vi "iitk.vi"() -> ()   [LabVIEW 2018]
uses:
  <vilib>/Waveform/WDTFileIO.llb/Read Waveform from File.vi
  <vilib>/express/express analysis/Spectral/Block/exnSpectralBlock spectral measurements peak poly.vi
  <vilib>/express/express analysis/Spectral/Block/exnSpectralBlock spectral measurements peak DDT.vi
  <vilib>/Waveform/WDTFileIO.llb/Export Waveforms To Spreadsheet File (1D).vi
  <vilib>/express/express analysis/Spectral/XNode/ExpressSpectralMeasurementsBlockNode.xnode
panel:
  in  "Operating Mode 3":T1(ring)=enum."Analyze Real-time"
  out "Orignal Signal 2":dynamicdata(graph)
  in  "Threshold 2":dbl=0.1
  out "Portion 2":dynamicdata(graph)
  in  "Portion Duration 2":i32=200
  out "Index 7":dbl
  out "Index 6":dbl
  out "Index 5":dbl
  out "Index 4":dbl
  out "dt1 2":dbl
  out "dt2 2":dbl
  out "dt3 2":dbl
  in  "Manual depth 2":dbl=4.3
  in  "Mode 2":T2(ring)=enum."Use Far Field"
  out "x 2":dbl format="%#_6f"
  out "y 2":dbl format="%#_6f"
  out "z 2":dbl
  in  "peak min 2":dbl=0.1
  out "ratio 8":dbl
  out "ratio 7":dbl
  out "ratio 6":dbl
  out "ratio 5":dbl
  out "amplitude 8":dbl
  out "amplitude 7":dbl
  out "amplitude 6":dbl
  out "amplitude 5":dbl
  out "yaw 2":dbl
  out "pitch 2":dbl
  out "Yaw Chart 2":dbl(graph)
  out "Freq Domain 2":dynamicdata(graph)
  out "Ratio at Index (%) 2":dbl
  in  "LPF Cut-Off 2":dbl=40000.0 caption="Lower Cut-Off"
  out "Selected Index 2":i32
  in  "method":bool
  in  "file path (dialog if empty)":path
  in  "Operating Mode 2":T1(ring)=enum."Analyze Real-time"
  out "Orignal Signal":dynamicdata(graph)
  in  "Threshold":dbl=0.1
  out "Portion":dynamicdata(graph)
  in  "Portion Duration":i32=200
  out "Index 0":dbl
  out "Index 1":dbl
  out "Index 2":dbl
  out "Index 3":dbl
  out "dt1":dbl
  out "dt2":dbl
  out "dt3":dbl
  in  "Manual depth":dbl=4.3
  in  "Mode":T2(ring)=enum."Use Far Field"
  out "x":dbl format="%#_6f"
  out "y":dbl format="%#_6f"
  out "z":dbl
  in  "peak min":dbl=0.1
  out "ratio":dbl
  out "ratio 2":dbl
  out "ratio 3":dbl
  out "ratio 4":dbl
  out "amplitude":dbl
  out "amplitude 2":dbl
  out "amplitude 3":dbl
  out "amplitude 4":dbl
  out "yaw":dbl
  out "pitch":dbl
  out "Yaw Chart":dbl(graph)
  out "Freq Domain":dynamicdata(graph)
  out "Ratio at Index (%)":dbl
  in  "LPF Cut-Off":dbl=40000.0 caption="Lower Cut-Off"
  out "Selected Index":i32
  in  "stop (F)":bool
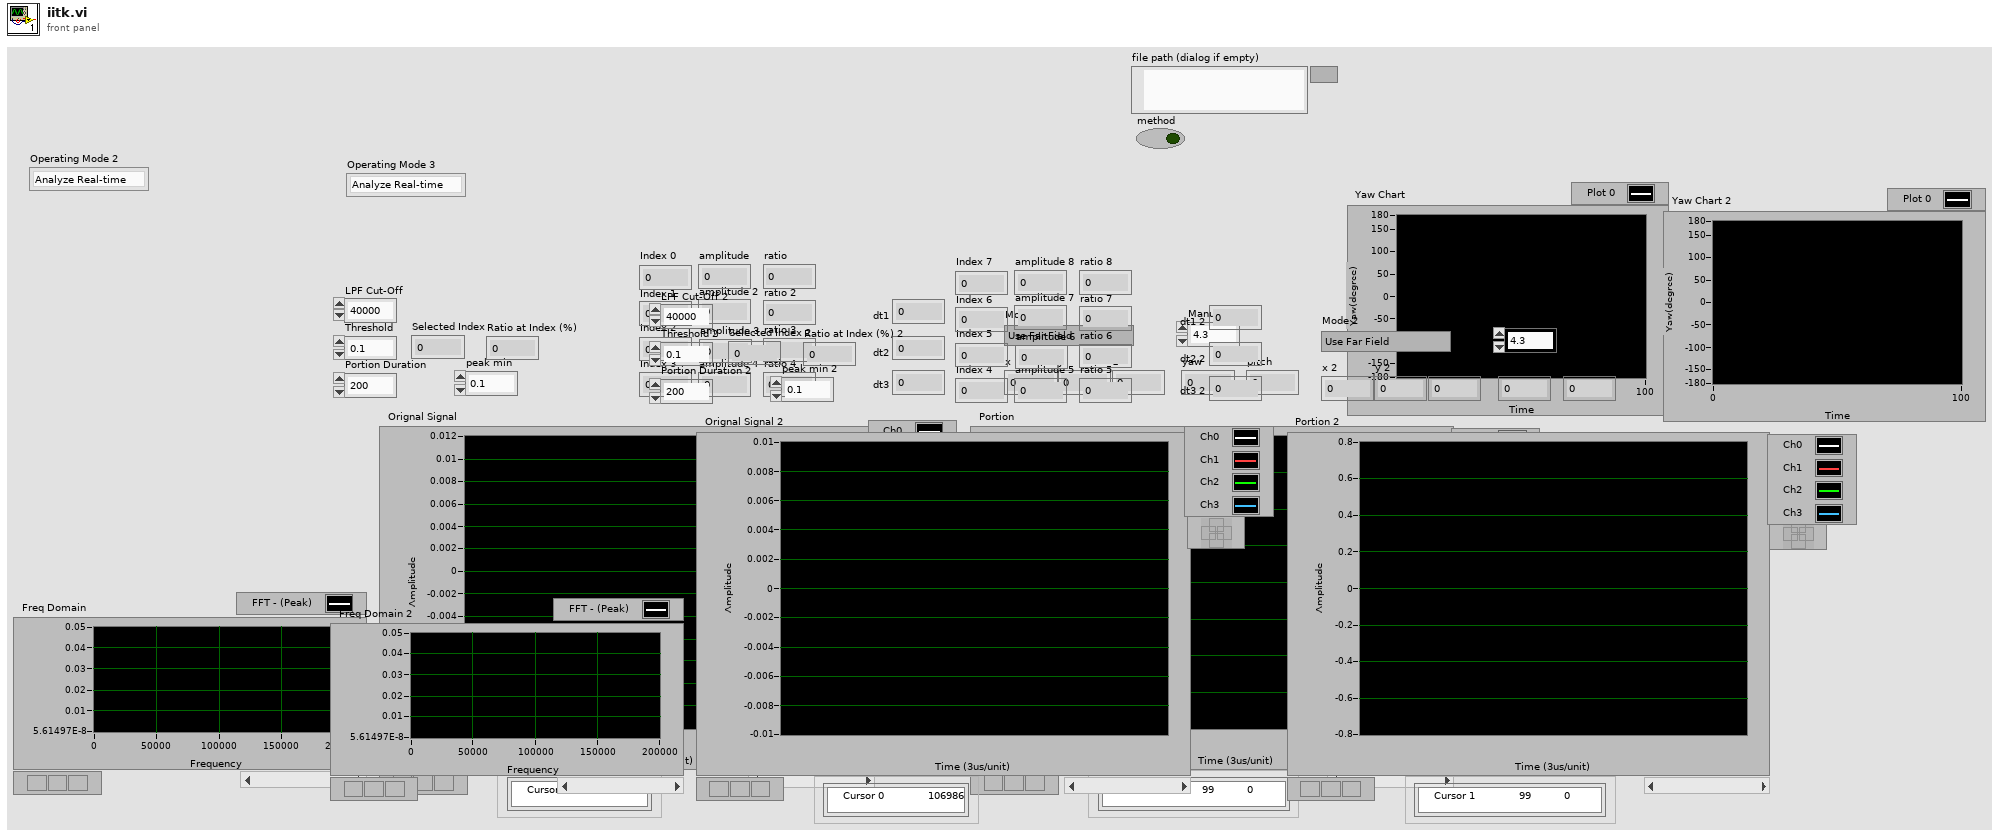
[diagram p1: front panel]
types:
  T1 = enum16{"Analyze From File", "Record Data", "Analyze Real-time"}
  T2 = enum16{"Use Near Field", "Use Far Field", "Send to ROS", "Far Field with 3 hydrophones"}
  T3 = cluster{"averaging mode":u16, "weighting mode":u16, "number of averages":u32}
  T4 = cluster{"dB On (F)":bool, "unwrap phase (F)":bool, "convert to degree (F)":bool}
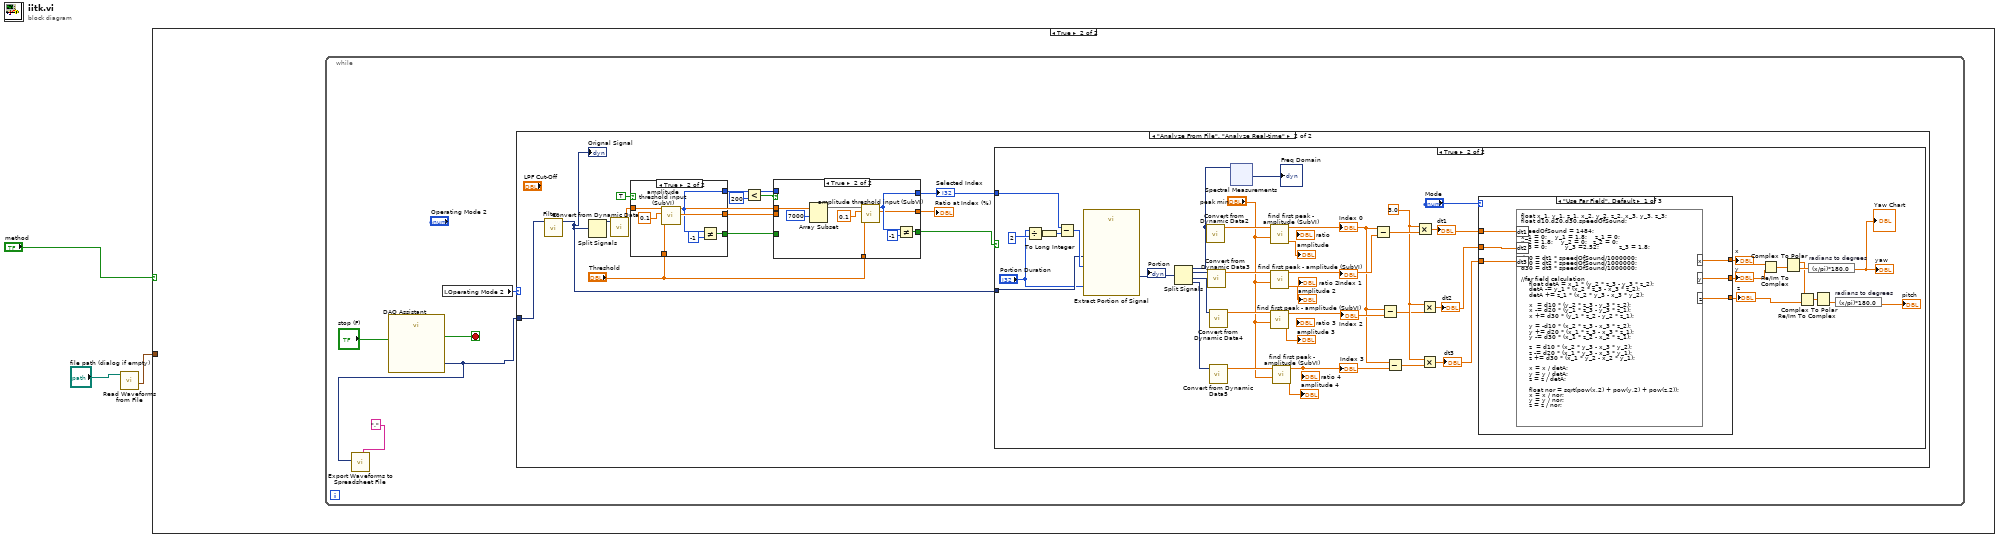
[diagram p0: block diagram]
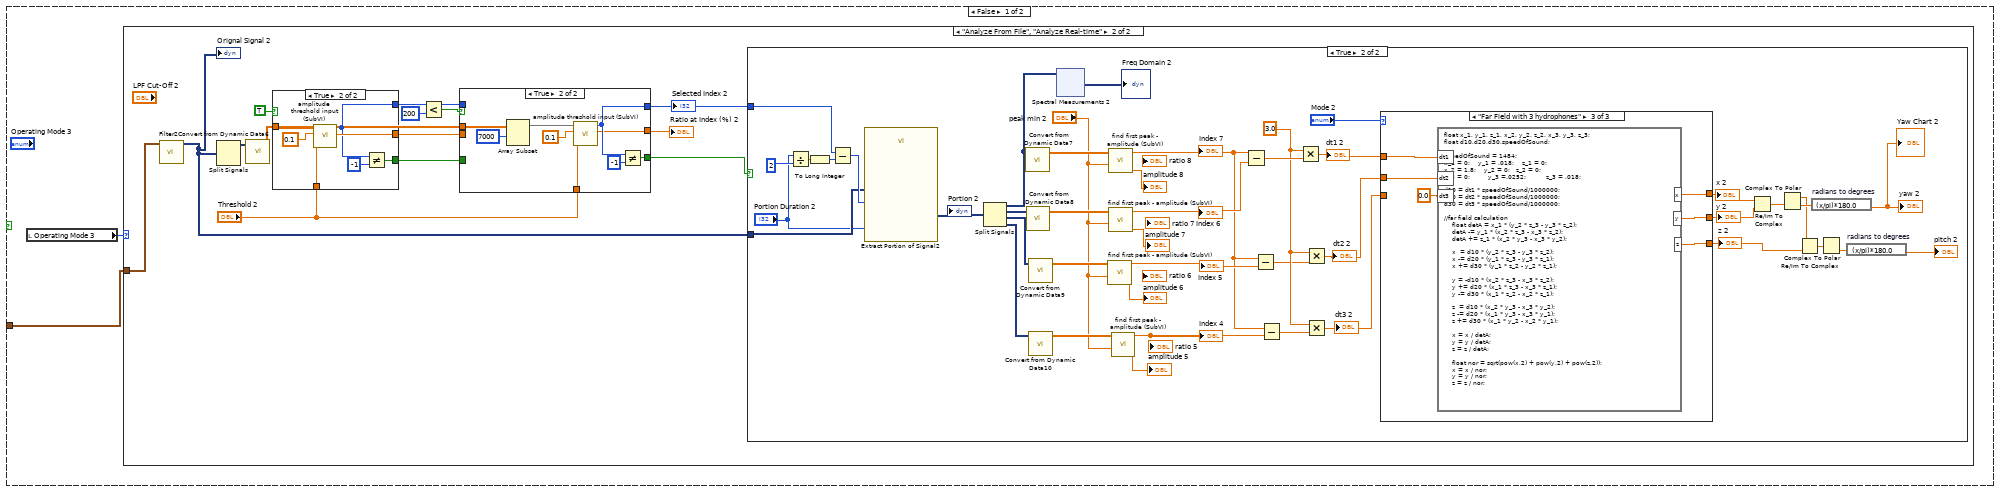
[diagram p2: hidden frame]
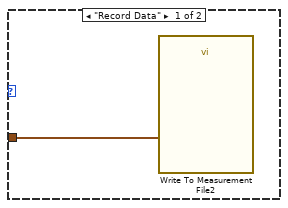
[diagram p3: hidden frame]
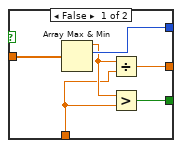
[diagram p5: hidden frame]
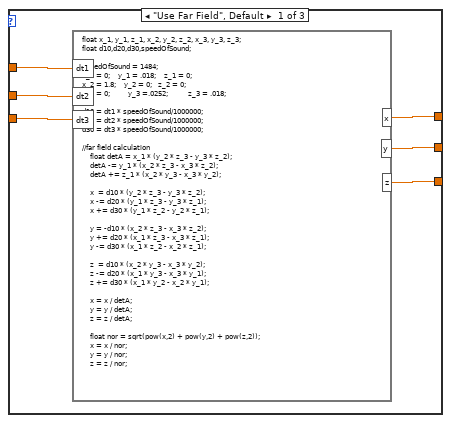
[diagram p7: hidden frame]
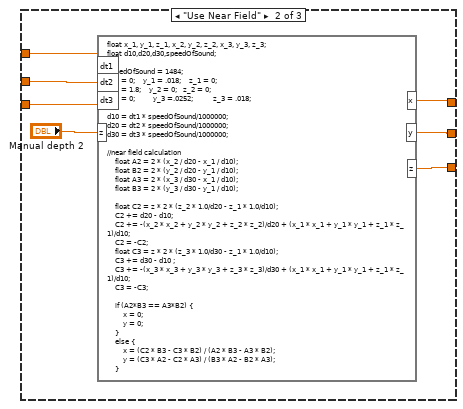
[diagram p8: hidden frame]
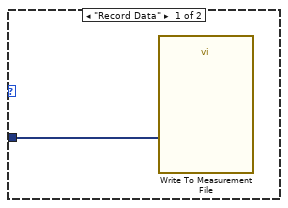
[diagram p9: hidden frame]
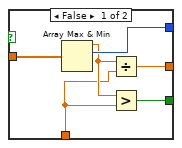
[diagram p11: hidden frame]
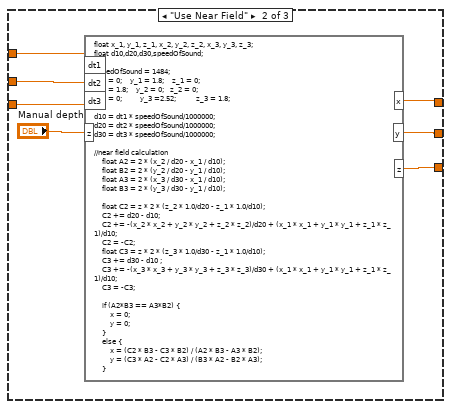
[diagram p13: hidden frame]
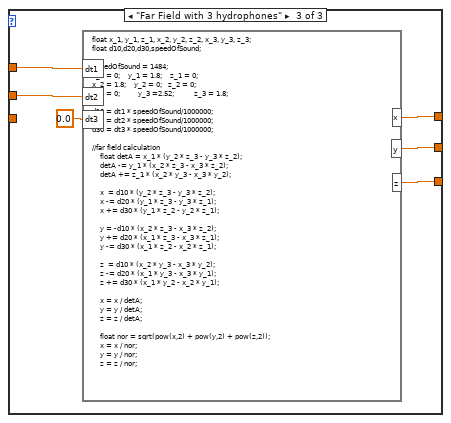
[diagram p14: hidden frame]
diagram:
  n1 = call-poly <vilib>:"Read Waveforms from File.vi"("file path (dialog if empty)"="file path (dialog if empty)") -> ("all waveforms in record"=w1:waveform(dbl)[])  [unwired: 5 in, 3 out]
  n2 = case shown="True" "method" {
    tunnel: w1 -> [w4 _]
    frame False {
      n3 = local read "Operating Mode 3"() -> (w5:T1)
      n4 = case shown="\"Analyze From File\", \"Analyze Real-time\"" w5 {
        tunnel: w4 -> [w6 w9]
        frame "Record Data" {
          n5 = call "Write To Measurement File2"("Signals"=w6) -> ()  [unwired: 16 in, 3 out]
        }
        frame "Analyze From File", "Analyze Real-time" {
          n6 = call "Filter2"("Signal"=w9) -> ("Filtered Signal"=w7:dynamicdata)  [unwired: 9 in, 1 out]
          "Orignal Signal 2" <- w7
          n7 = Split Signals(w7) -> (w8:dynamicdata)  [unwired: 4 in, 3 out]
          n8 = call "Convert from Dynamic Data6"("Dynamic Data Type"=w8) -> ("Array"=w15:dbl[])  [unwired: 3 in]
          n9 = case shown="True" TRUE {
            tunnel: w15 -> [w38 w45]
            tunnel: [w35 w42] -> w16
            tunnel: [w36 w41] -> w11
            tunnel: [w37 w40] -> w19
            tunnel: "Threshold 2" -> [w33 w39]
            frame False {
              n10 = Array Max & Min(array=w38) -> (max value=w34:dbl, max index (indices)=w36:i32)  [unwired: 2 out]
              n11 = Divide(x=w34, y=w33) -> (x/y=w35:dbl)
              n12 = Greater?(x=w34, y=w33) -> (0:w37:bool)
            }
            frame True {
              n13 = call "amplitude threshold input (SubVI).vi"("threshold"=w39, "%max amplitude"=0.1, "Array"=w45) -> ("actual ratio (%)"=w42:dbl, "Index"=w41:i32)  [unwired: 7 in]
              n14 = Not Equal?(x=w41, y=-1) -> (x != y?=w40:bool)
            }
          }
          n15 = Less?(x=w11, y=200) -> (x < y?=w17:bool)
          n16 = case shown="True" w17 {
            tunnel: w19 -> [w23 _]
            tunnel: w16 -> [w21 _]
            tunnel: w15 -> [_ w32]
            tunnel: "Threshold 2" -> [_ w27]
            tunnel: [w23 w26] -> w13
            tunnel: [w22 w25] -> w10
            tunnel: [w21 w24] -> w12
            tunnel: w11 -> [w22 _]
            frame False {
            }
            frame True {
              n17 = Array Subset(array=w32, index=7000) -> (w28:dbl[])  [unwired: 1 in]
              n18 = call "amplitude threshold input (SubVI).vi"("threshold"=w27, "%max amplitude"=0.1, "Array"=w28) -> ("actual ratio (%)"=w24:dbl, "Index"=w25:i32)  [unwired: 7 in]
              n19 = Not Equal?(x=w25, y=-1) -> (x != y?=w26:bool)
            }
          }
          "Ratio at Index (%) 2" <- w12
          "Selected Index 2" <- w10
          n20 = case shown="True" w13 {
            tunnel: w7 -> [_ w86]
            tunnel: w10 -> [_ w52]
            frame False {
            }
            frame True {
              w82 = 3.0 ("x")
              n21 = Divide(x="Portion Duration 2", y=2) -> (x/y=w56:dbl)
              n22 = To Long Integer(number=w56) -> (32bit integer=w55:i32)
              n23 = Subtract(x=w52, y=w55) -> (x-y=w89:i32)
              n24 = call "Extract Portion of Signal2"("Samples"="Portion Duration 2", "Begin Sample"=w89, "Signals"=w86) -> ("Section"=w85:dynamicdata)  [unwired: 7 in, 1 out]
              "Portion 2" <- w85
              n25 = Split Signals(w85) -> (w46:dynamicdata, w88:dynamicdata, w87:dynamicdata, w84:dynamicdata)  [unwired: 4 in]
              n26 = call "Convert from Dynamic Data7"("Dynamic Data Type"=w46) -> ("Array"=w77:dbl[])  [unwired: 3 in]
              n27 = call "Convert from Dynamic Data8"("Dynamic Data Type"=w88) -> ("Array"=w76:dbl[])  [unwired: 3 in]
              n28 = call "Convert from Dynamic Data9"("Dynamic Data Type"=w87) -> ("Array"=w75:dbl[])  [unwired: 3 in]
              n29 = call "Convert from Dynamic Data10"("Dynamic Data Type"=w84) -> ("Array"=w74:dbl[])  [unwired: 3 in]
              n30 = xnode "Spectral Measurements 2"("Signals"=w46) -> ("FFT - (Peak)"=→"Freq Domain 2":dynamicdata)  [unwired: 1 in, 2 out]
              n31 = call "find first peak - amplitude (SubVI).vi"("threshold ratio"="peak min 2", "Array"=w75) -> ("Peak threshold"=→"amplitude 6":dbl, "Index"=w72:dbl)  [unwired: 5 in, 3 out]
              "Index 5" <- w72
              n32 = call "find first peak - amplitude (SubVI).vi"("threshold ratio"="peak min 2", "Array"=w77) -> ("Peak threshold"=→"amplitude 8":dbl, "Index"=w71:dbl)  [unwired: 5 in, 3 out]
              "Index 7" <- w71
              n33 = call "find first peak - amplitude (SubVI).vi"("threshold ratio"="peak min 2", "Array"=w76) -> ("Peak threshold"=→"amplitude 7":dbl, "Index"=w73:dbl)  [unwired: 5 in, 3 out]
              "Index 6" <- w73
              n34 = call "find first peak - amplitude (SubVI).vi"("threshold ratio"="peak min 2", "Array"=w74) -> ("Peak threshold"=→"amplitude 5":dbl, "Index"=w70:dbl)  [unwired: 5 in, 3 out]
              "Index 4" <- w70
              n35 = Subtract(x=w71, y=w73) -> (x-y=w83:dbl)
              n36 = Subtract(x=w71, y=w72) -> (x-y=w81:dbl)
              n37 = Subtract(x=w71, y=w70) -> (x-y=w80:dbl)
              n38 = Multiply(x=w82, y=w83) -> (x*y=w59:dbl)
              "dt1 2" <- w59
              n39 = Multiply(x=w82, y=w81) -> (x*y=w79:dbl)
              "dt2 2" <- w79
              n40 = Multiply(x=w82, y=w80) -> (x*y=w58:dbl)
              "dt3 2" <- w58
              n41 = case shown="\"Far Field with 3 hydrophones\"" "Mode 2" {
                tunnel: w59 -> [w105 w112 w118]
                tunnel: w79 -> [w104 w111 w117]
                tunnel: [w103 w110 w115] -> w66
                tunnel: [w102 w109 w114] -> w65
                tunnel: [w101 w108 w113] -> w64
                tunnel: w58 -> [w100 w106 _]
                frame "Use Far Field", Default {
                  n42 = formula code="float x_1, y_1, z_1, x_2, y_2, z_2, x_3, y_3, z_3;\nfloat d10,d20,d30,speedOfSound;\n\nspeedOfSound = 1484;\nx_1 = 0;    y_1 = .018;    z_1 = 0;\nx_2 = 1.8;    y_2 = 0;   z_2 = 0;\nx_3 = 0;         y_3 =.0252;          z_3 = .018;\n\nd10 = dt1 * speedOfSound/1000000;\nd20 = dt2 * speedOfSound/1000000;\nd30 = dt3 * speedOfSound/1000000;\n\n//far field calculation\n    float detA = x_1 * (y_2 * z_3 - y_3 * z_2);\n    detA -= y_1 * (x_2 * z_3 - x_3 * z_2);\n    detA += z_1 * (x_2 * y_3 - x_3 * y_2);\n\n    x  = d10 * (y_2 * z_3 - y_3 * z_2);\n    x -= d20 * (y_1 * z_3 - y_3 * z_1);\n    x += d30 * (y_1 * z_2 - y_2 * z_1);\n\n    y = -d10 * (x_2 * z_3 - x_3 * z_2);\n    y += d20 * (x_1 * z_3 - x_3 * z_1);\n    y -= d30 * (x_1 * z_2 - x_2 * z_1);\n\n    z  = d10 * (x_2 * y_3 - x_3 * y_2);\n    z -= d20 * (x_1 * y_3 - x_3 * y_1);\n    z += d30 * (x_1 * y_2 - x_2 * y_1);\n\n    x = x / detA;\n    y = y / detA;\n    z = z / detA;\n\n    float nor = sqrt(pow(x,2) + pow(y,2) + pow(z,2));\n    x = x / nor;\n    y = y / nor;\n    z = z / nor;"("dt1"=w105, "dt2"=w104, "dt3"=w100) -> ("x"=w103:dbl, "y"=w102:dbl, "z"=w101:dbl)
                }
                frame "Use Near Field" {
                  n43 = formula code="float x_1, y_1, z_1, x_2, y_2, z_2, x_3, y_3, z_3;\nfloat d10,d20,d30,speedOfSound;\n\nspeedOfSound = 1484;\nx_1 = 0;    y_1 = .018;    z_1 = 0;\nx_2 = 1.8;    y_2 = 0;   z_2 = 0;\nx_3 = 0;         y_3 =.0252;          z_3 = .018;\n\nd10 = dt1 * speedOfSound/1000000;\nd20 = dt2 * speedOfSound/1000000;\nd30 = dt3 * speedOfSound/1000000;\n\n//near field calculation\n    float A2 = 2 * (x_2 / d20 - x_1 / d10);\n    float B2 = 2 * (y_2 / d20 - y_1 / d10);\n    float A3 = 2 * (x_3 / d30 - x_1 / d10);\n    float B3 = 2 * (y_3 / d30 - y_1 / d10);\n    \n    float C2 = z * 2 * (z_2 * 1.0/d20 - z_1 * 1.0/d10);\n    C2 += d20 - d10;\n    C2 += -(x_2 * x_2 + y_2 * y_2 + z_2 * z_2)/d20 + (x_1 * x_1 + y_1 * y_1 + z_1 * z_1)/d10;\n    C2 = -C2;\n    float C3 = z * 2 * (z_3 * 1.0/d30 - z_1 * 1.0/d10);\n    C3 += d30 - d10 ;\n    C3 += -(x_3 * x_3 + y_3 * y_3 + z_3 * z_3)/d30 + (x_1 * x_1 + y_1 * y_1 + z_1 * z_1)/d10;\n    C3 = -C3;\n\n    if (A2*B3 == A3*B2) {\n        x = 0;\n        y = 0;\n    }\n    else {\n        x = (C2 * B3 - C3 * B2) / (A2 * B3 - A3 * B2);\n        y = (C3 * A2 - C2 * A3) / (B3 * A2 - B2 * A3);\n    }"("dt1"=w112, "dt2"=w111, "dt3"=w106, "z"="Manual depth 2") -> ("x"=w110:dbl, "y"=w109:dbl, "z"=w108:dbl)
                }
                frame "Far Field with 3 hydrophones" {
                  n44 = formula code="float x_1, y_1, z_1, x_2, y_2, z_2, x_3, y_3, z_3;\nfloat d10,d20,d30,speedOfSound;\n\nspeedOfSound = 1484;\nx_1 = 0;    y_1 = .018;    z_1 = 0;\nx_2 = 1.8;    y_2 = 0;   z_2 = 0;\nx_3 = 0;         y_3 =.0252;          z_3 = .018;\n\nd10 = dt1 * speedOfSound/1000000;\nd20 = dt2 * speedOfSound/1000000;\nd30 = dt3 * speedOfSound/1000000;\n\n//far field calculation\n    float detA = x_1 * (y_2 * z_3 - y_3 * z_2);\n    detA -= y_1 * (x_2 * z_3 - x_3 * z_2);\n    detA += z_1 * (x_2 * y_3 - x_3 * y_2);\n\n    x  = d10 * (y_2 * z_3 - y_3 * z_2);\n    x -= d20 * (y_1 * z_3 - y_3 * z_1);\n    x += d30 * (y_1 * z_2 - y_2 * z_1);\n\n    y = -d10 * (x_2 * z_3 - x_3 * z_2);\n    y += d20 * (x_1 * z_3 - x_3 * z_1);\n    y -= d30 * (x_1 * z_2 - x_2 * z_1);\n\n    z  = d10 * (x_2 * y_3 - x_3 * y_2);\n    z -= d20 * (x_1 * y_3 - x_3 * y_1);\n    z += d30 * (x_1 * y_2 - x_2 * y_1);\n\n    x = x / detA;\n    y = y / detA;\n    z = z / detA;\n\n    float nor = sqrt(pow(x,2) + pow(y,2) + pow(z,2));\n    x = x / nor;\n    y = y / nor;\n    z = z / nor;"("dt1"=w118, "dt2"=w117, "dt3"=0.0 ("input variable")) -> ("x"=w115:dbl, "y"=w114:dbl, "z"=w113:dbl)
                }
              }
              "x 2" <- w66
              "y 2" <- w65
              "z 2" <- w64
              n45 = Re/Im To Complex(1:w65, 2:w66) -> (0:w68:cdb)
              n46 = Complex To Polar(r * e^(i*theta)=w68) -> (r=w63:dbl, theta=w67:dbl)
              n47 = Re/Im To Complex(1:w64, 2:w63) -> (0:w62:cdb)
              n48 = expression code="(x/pi)*180.0" "radians to degrees"(w67) -> (→"yaw 2" →"Yaw Chart 2":dbl)
              n49 = Complex To Polar(r * e^(i*theta)=w62) -> (theta=w60:dbl)  [unwired: 1 out]
              n50 = expression code="(x/pi)*180.0" "radians to degrees"(w60) -> (→"pitch 2":dbl)
            }
          }
        }
      }
    }
    frame True {
      n51 = while {
        stop <- w123 stop-if-true
        n52 = call "DAQ Assistant"("stop (F)"="stop (F)") -> ("data"=w119:dynamicdata, "stopped"=w123:bool)  [unwired: 15 in, 2 out]
        n53 = call-poly <vilib>:"Export Waveforms to Spreadsheet File.vi"("delimiter (Tab)"=".", "waveforms"=w119) -> ()  [unwired: 8 in, 2 out]
        n54 = local read "Operating Mode 2"() -> (w121:T1)
        n55 = case shown="\"Analyze From File\", \"Analyze Real-time\"" w121 {
          tunnel: w119 -> [w124 w127]
          frame "Record Data" {
            n56 = call "Write To Measurement File"("Signals"=w124) -> ()  [unwired: 16 in, 3 out]
          }
          frame "Analyze From File", "Analyze Real-time" {
            n57 = call "Filter"("Signal"=w127) -> ("Filtered Signal"=w125:dynamicdata)  [unwired: 9 in, 1 out]
            "Orignal Signal" <- w125
            n58 = Split Signals(w125) -> (w126:dynamicdata)  [unwired: 4 in, 3 out]
            n59 = call "Convert from Dynamic Data"("Dynamic Data Type"=w126) -> ("Array"=w133:dbl[])  [unwired: 3 in]
            n60 = case shown="True" TRUE {
              tunnel: w133 -> [w156 w163]
              tunnel: [w153 w160] -> w134
              tunnel: [w154 w159] -> w129
              tunnel: [w155 w158] -> w137
              tunnel: "Threshold" -> [w151 w157]
              frame False {
                n61 = Array Max & Min(array=w156) -> (max value=w152:dbl, max index (indices)=w154:i32)  [unwired: 2 out]
                n62 = Divide(x=w152, y=w151) -> (x/y=w153:dbl)
                n63 = Greater?(x=w152, y=w151) -> (0:w155:bool)
              }
              frame True {
                n64 = call "amplitude threshold input (SubVI).vi"("threshold"=w157, "%max amplitude"=0.1, "Array"=w163) -> ("actual ratio (%)"=w160:dbl, "Index"=w159:i32)  [unwired: 7 in]
                n65 = Not Equal?(x=w159, y=-1) -> (x != y?=w158:bool)
              }
            }
            n66 = Less?(x=w129, y=200) -> (x < y?=w135:bool)
            n67 = case shown="True" w135 {
              tunnel: w137 -> [w141 _]
              tunnel: w134 -> [w139 _]
              tunnel: w133 -> [_ w150]
              tunnel: "Threshold" -> [_ w145]
              tunnel: [w141 w144] -> w131
              tunnel: [w140 w143] -> w128
              tunnel: [w139 w142] -> w130
              tunnel: w129 -> [w140 _]
              frame False {
              }
              frame True {
                n68 = Array Subset(array=w150, index=7000) -> (w146:dbl[])  [unwired: 1 in]
                n69 = call "amplitude threshold input (SubVI).vi"("threshold"=w145, "%max amplitude"=0.1, "Array"=w146) -> ("actual ratio (%)"=w142:dbl, "Index"=w143:i32)  [unwired: 7 in]
                n70 = Not Equal?(x=w143, y=-1) -> (x != y?=w144:bool)
              }
            }
            "Ratio at Index (%)" <- w130
            "Selected Index" <- w128
            n71 = case shown="True" w131 {
              tunnel: w125 -> [_ w204]
              tunnel: w128 -> [_ w170]
              frame False {
              }
              frame True {
                w200 = 3.0 ("x")
                n72 = Divide(x="Portion Duration", y=2) -> (x/y=w174:dbl)
                n73 = To Long Integer(number=w174) -> (32bit integer=w173:i32)
                n74 = Subtract(x=w170, y=w173) -> (x-y=w207:i32)
                n75 = call "Extract Portion of Signal"("Samples"="Portion Duration", "Begin Sample"=w207, "Signals"=w204) -> ("Section"=w203:dynamicdata)  [unwired: 7 in, 1 out]
                "Portion" <- w203
                n76 = Split Signals(w203) -> (w164:dynamicdata, w206:dynamicdata, w205:dynamicdata, w202:dynamicdata)  [unwired: 4 in]
                n77 = call "Convert from Dynamic Data2"("Dynamic Data Type"=w164) -> ("Array"=w195:dbl[])  [unwired: 3 in]
                n78 = call "Convert from Dynamic Data3"("Dynamic Data Type"=w206) -> ("Array"=w194:dbl[])  [unwired: 3 in]
                n79 = call "Convert from Dynamic Data4"("Dynamic Data Type"=w205) -> ("Array"=w193:dbl[])  [unwired: 3 in]
                n80 = call "Convert from Dynamic Data5"("Dynamic Data Type"=w202) -> ("Array"=w192:dbl[])  [unwired: 3 in]
                n81 = xnode "Spectral Measurements"("Signals"=w164) -> ("FFT - (Peak)"=→"Freq Domain":dynamicdata)  [unwired: 1 in, 2 out]
                n82 = call "find first peak - amplitude (SubVI).vi"("threshold ratio"="peak min", "Array"=w193) -> ("Peak threshold"=→"amplitude 3":dbl, "Index"=w190:dbl)  [unwired: 5 in, 3 out]
                "Index 2" <- w190
                n83 = call "find first peak - amplitude (SubVI).vi"("threshold ratio"="peak min", "Array"=w195) -> ("Peak threshold"=→"amplitude":dbl, "Index"=w189:dbl)  [unwired: 5 in, 3 out]
                "Index 0" <- w189
                n84 = call "find first peak - amplitude (SubVI).vi"("threshold ratio"="peak min", "Array"=w194) -> ("Peak threshold"=→"amplitude 2":dbl, "Index"=w191:dbl)  [unwired: 5 in, 3 out]
                "Index 1" <- w191
                n85 = call "find first peak - amplitude (SubVI).vi"("threshold ratio"="peak min", "Array"=w192) -> ("Peak threshold"=→"amplitude 4":dbl, "Index"=w188:dbl)  [unwired: 5 in, 3 out]
                "Index 3" <- w188
                n86 = Subtract(x=w189, y=w191) -> (x-y=w201:dbl)
                n87 = Subtract(x=w189, y=w190) -> (x-y=w199:dbl)
                n88 = Subtract(x=w189, y=w188) -> (x-y=w198:dbl)
                n89 = Multiply(x=w200, y=w201) -> (x*y=w177:dbl)
                "dt1" <- w177
                n90 = Multiply(x=w200, y=w199) -> (x*y=w197:dbl)
                "dt2" <- w197
                n91 = Multiply(x=w200, y=w198) -> (x*y=w176:dbl)
                "dt3" <- w176
                n92 = case shown="\"Use Far Field\", Default" "Mode" {
                  tunnel: w177 -> [w223 w230 w236]
                  tunnel: w197 -> [w222 w229 w235]
                  tunnel: [w221 w228 w233] -> w184
                  tunnel: [w220 w227 w232] -> w183
                  tunnel: [w219 w226 w231] -> w182
                  tunnel: w176 -> [w218 w224 _]
                  frame "Use Far Field", Default {
                    n93 = formula code="float x_1, y_1, z_1, x_2, y_2, z_2, x_3, y_3, z_3;\nfloat d10,d20,d30,speedOfSound;\n\nspeedOfSound = 1484;\nx_1 = 0;    y_1 = 1.8;    z_1 = 0;\nx_2 = 1.8;    y_2 = 0;   z_2 = 0;\nx_3 = 0;         y_3 =2.52;          z_3 = 1.8;\n\nd10 = dt1 * speedOfSound/1000000;\nd20 = dt2 * speedOfSound/1000000;\nd30 = dt3 * speedOfSound/1000000;\n\n//far field calculation\n    float detA = x_1 * (y_2 * z_3 - y_3 * z_2);\n    detA -= y_1 * (x_2 * z_3 - x_3 * z_2);\n    detA += z_1 * (x_2 * y_3 - x_3 * y_2);\n\n    x  = d10 * (y_2 * z_3 - y_3 * z_2);\n    x -= d20 * (y_1 * z_3 - y_3 * z_1);\n    x += d30 * (y_1 * z_2 - y_2 * z_1);\n\n    y = -d10 * (x_2 * z_3 - x_3 * z_2);\n    y += d20 * (x_1 * z_3 - x_3 * z_1);\n    y -= d30 * (x_1 * z_2 - x_2 * z_1);\n\n    z  = d10 * (x_2 * y_3 - x_3 * y_2);\n    z -= d20 * (x_1 * y_3 - x_3 * y_1);\n    z += d30 * (x_1 * y_2 - x_2 * y_1);\n\n    x = x / detA;\n    y = y / detA;\n    z = z / detA;\n\n    float nor = sqrt(pow(x,2) + pow(y,2) + pow(z,2));\n    x = x / nor;\n    y = y / nor;\n    z = z / nor;"("dt1"=w223, "dt2"=w222, "dt3"=w218) -> ("x"=w221:dbl, "y"=w220:dbl, "z"=w219:dbl)
                  }
                  frame "Use Near Field" {
                    n94 = formula code="float x_1, y_1, z_1, x_2, y_2, z_2, x_3, y_3, z_3;\nfloat d10,d20,d30,speedOfSound;\n\nspeedOfSound = 1484;\nx_1 = 0;    y_1 = 1.8;    z_1 = 0;\nx_2 = 1.8;    y_2 = 0;   z_2 = 0;\nx_3 = 0;         y_3 =2.52;          z_3 = 1.8;\n\nd10 = dt1 * speedOfSound/1000000;\nd20 = dt2 * speedOfSound/1000000;\nd30 = dt3 * speedOfSound/1000000;\n\n//near field calculation\n    float A2 = 2 * (x_2 / d20 - x_1 / d10);\n    float B2 = 2 * (y_2 / d20 - y_1 / d10);\n    float A3 = 2 * (x_3 / d30 - x_1 / d10);\n    float B3 = 2 * (y_3 / d30 - y_1 / d10);\n    \n    float C2 = z * 2 * (z_2 * 1.0/d20 - z_1 * 1.0/d10);\n    C2 += d20 - d10;\n    C2 += -(x_2 * x_2 + y_2 * y_2 + z_2 * z_2)/d20 + (x_1 * x_1 + y_1 * y_1 + z_1 * z_1)/d10;\n    C2 = -C2;\n    float C3 = z * 2 * (z_3 * 1.0/d30 - z_1 * 1.0/d10);\n    C3 += d30 - d10 ;\n    C3 += -(x_3 * x_3 + y_3 * y_3 + z_3 * z_3)/d30 + (x_1 * x_1 + y_1 * y_1 + z_1 * z_1)/d10;\n    C3 = -C3;\n\n    if (A2*B3 == A3*B2) {\n        x = 0;\n        y = 0;\n    }\n    else {\n        x = (C2 * B3 - C3 * B2) / (A2 * B3 - A3 * B2);\n        y = (C3 * A2 - C2 * A3) / (B3 * A2 - B2 * A3);\n    }"("dt1"=w230, "dt2"=w229, "dt3"=w224, "z"="Manual depth") -> ("x"=w228:dbl, "y"=w227:dbl, "z"=w226:dbl)
                  }
                  frame "Far Field with 3 hydrophones" {
                    n95 = formula code="float x_1, y_1, z_1, x_2, y_2, z_2, x_3, y_3, z_3;\nfloat d10,d20,d30,speedOfSound;\n\nspeedOfSound = 1484;\nx_1 = 0;    y_1 = 1.8;    z_1 = 0;\nx_2 = 1.8;    y_2 = 0;   z_2 = 0;\nx_3 = 0;         y_3 =2.52;          z_3 = 1.8;\n\nd10 = dt1 * speedOfSound/1000000;\nd20 = dt2 * speedOfSound/1000000;\nd30 = dt3 * speedOfSound/1000000;\n\n//far field calculation\n    float detA = x_1 * (y_2 * z_3 - y_3 * z_2);\n    detA -= y_1 * (x_2 * z_3 - x_3 * z_2);\n    detA += z_1 * (x_2 * y_3 - x_3 * y_2);\n\n    x  = d10 * (y_2 * z_3 - y_3 * z_2);\n    x -= d20 * (y_1 * z_3 - y_3 * z_1);\n    x += d30 * (y_1 * z_2 - y_2 * z_1);\n\n    y = -d10 * (x_2 * z_3 - x_3 * z_2);\n    y += d20 * (x_1 * z_3 - x_3 * z_1);\n    y -= d30 * (x_1 * z_2 - x_2 * z_1);\n\n    z  = d10 * (x_2 * y_3 - x_3 * y_2);\n    z -= d20 * (x_1 * y_3 - x_3 * y_1);\n    z += d30 * (x_1 * y_2 - x_2 * y_1);\n\n    x = x / detA;\n    y = y / detA;\n    z = z / detA;\n\n    float nor = sqrt(pow(x,2) + pow(y,2) + pow(z,2));\n    x = x / nor;\n    y = y / nor;\n    z = z / nor;"("dt1"=w236, "dt2"=w235, "dt3"=0.0 ("input variable")) -> ("x"=w233:dbl, "y"=w232:dbl, "z"=w231:dbl)
                  }
                }
                "x" <- w184
                "y" <- w183
                "z" <- w182
                n96 = Re/Im To Complex(1:w183, 2:w184) -> (0:w186:cdb)
                n97 = Complex To Polar(r * e^(i*theta)=w186) -> (r=w181:dbl, theta=w185:dbl)
                n98 = Re/Im To Complex(1:w182, 2:w181) -> (0:w180:cdb)
                n99 = expression code="(x/pi)*180.0" "radians to degrees"(w185) -> (→"yaw" →"Yaw Chart":dbl)
                n100 = Complex To Polar(r * e^(i*theta)=w180) -> (theta=w178:dbl)  [unwired: 1 out]
                n101 = expression code="(x/pi)*180.0" "radians to degrees"(w178) -> (→"pitch":dbl)
              }
            }
          }
        }
      }
    }
  }
